vi "Read Legend Plot Visibility.vi"(9 "WaveformChart in":refnum<class "WaveformGraph.lvclass">) -> (3 "WaveformChart out":refnum<class "WaveformGraph.lvclass">, 4 "Legend Plot Visibility":bool)   [LabVIEW 2014, in "WaveformGraph.lvclass"]
uses:
  WaveformGraph.lvclass
  WaveformGraph.lvclass/WaveformGraph.ctl
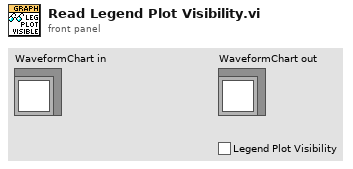
[diagram p1: front panel]
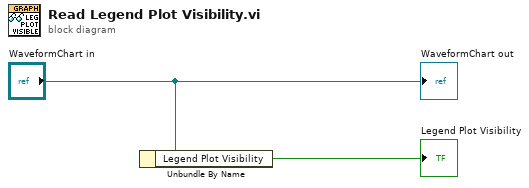
[diagram p0: block diagram]
diagram:
  n1 = Unbundle By Name("WaveformChart in") -> ("Legend Plot Visibility"=→"Legend Plot Visibility":bool)
  "WaveformChart out" <- "WaveformChart in"
